vi "Save File to LABVIEW Menu.vi"(8 "错误输入":errorcluster, 10 "Sub Dir":string="\\Custom", 11 "Select VI":path) -> (0 "错误输出":errorcluster)   [LabVIEW 2012]
panel:
  in  "Dir":string(combo)="wizard"
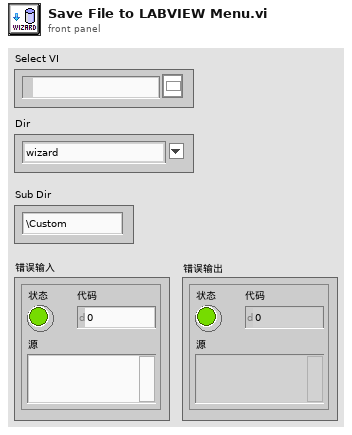
[diagram p1: front panel]
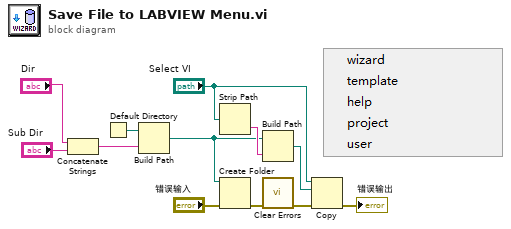
[diagram p0: block diagram]
diagram:
  n1 = Concatenate Strings("Dir", "Sub Dir") -> (w4:string)
  n2 = Default Directory() -> (w12:path)
  n3 = Build Path(base path=w12, name or relative path=w4) -> (appended path=w2:path)
  n4 = Strip Path(path="Select VI") -> (name=w11:string)  [unwired: 1 out]
  n5 = Create Folder(path (use dialog)=w2, error in="错误输入") -> (error out=w7:errorcluster)  [unwired: 1 in, 2 out]
  n6 = Build Path(base path=w2, name or relative path=w11) -> (appended path=w8:path)
  n7 = call <vilib>:"Clear Errors.vi"("error in (no error)"=w7) -> ("error out"=w3:errorcluster)  [unwired: 6 in]
  n8 = Copy(8:w3, 10:w8, 11:"Select VI") -> (0:→"错误输出":errorcluster)  [unwired: 2 in, 2 out]
